vi "Write Test Sequence.vi"(8 "error in (no error)":errorcluster, 10 "Test Sequence":T1, 11 "NI DAQmx in":refnum<class "NI DAQmx.lvclass">) -> (0 "error out":errorcluster, 3 "NI DAQmx out":refnum<class "NI DAQmx.lvclass">)   [LabVIEW 2020, in "NI DAQmx.lvclass"]
uses:
  NI DAQmx.lvclass
  NI DAQmx.lvclass/NI DAQmx.ctl
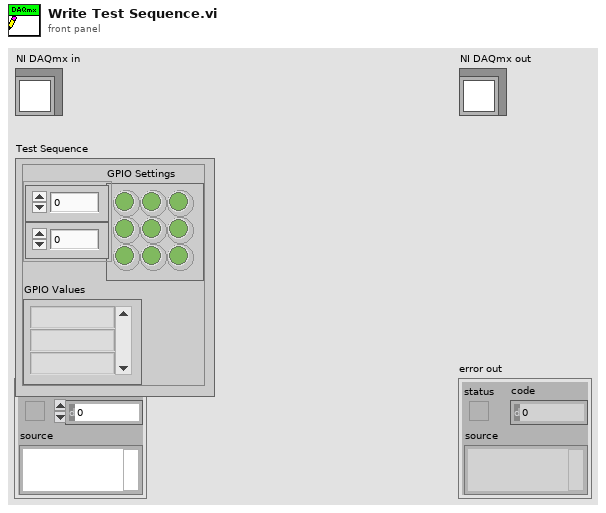
[diagram p1: front panel]
types:
  T1 = cluster{"GPIO Settings":bool[][], "GPIO Values":string[]}
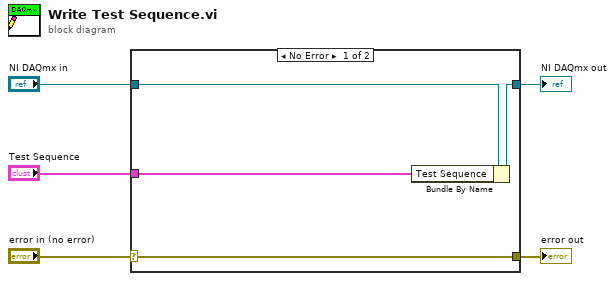
[diagram p0: block diagram]
diagram:
  n1 = case shown="No Error" "error in (no error)" {
    selector: "error in (no error)" -> [w9 w10]
    tunnel: [w9 w10] -> w4
    tunnel: [w7 w11] -> w2
    tunnel: "NI DAQmx in" -> [w8 w11]
    tunnel: "Test Sequence" -> [w6 _]
    frame No Error {
      n2 = Bundle By Name(cluster=w8, "Test Sequence"=w6) -> (w7:refnum<class "NI DAQmx.lvclass">)
    }
    frame Error {
    }
  }
  "error out" <- w4
  "NI DAQmx out" <- w2
